vi "DP-Show Noise Floor Data.vi"(1 "Listbox Refnum":refnum<vi>, 9 "Names":string[](array[string]), 11 "error in":errorcluster, 13 "Noise floor data":dbl[][](array[numeric])) -> (15 "error out":errorcluster)   [LabVIEW 2020]
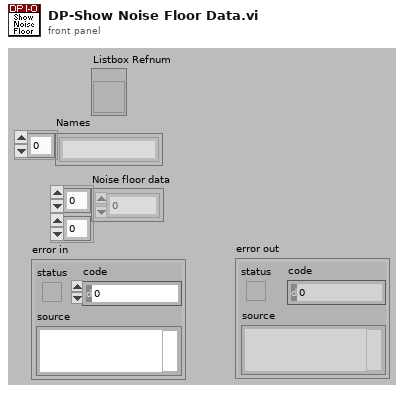
[diagram p1: front panel]
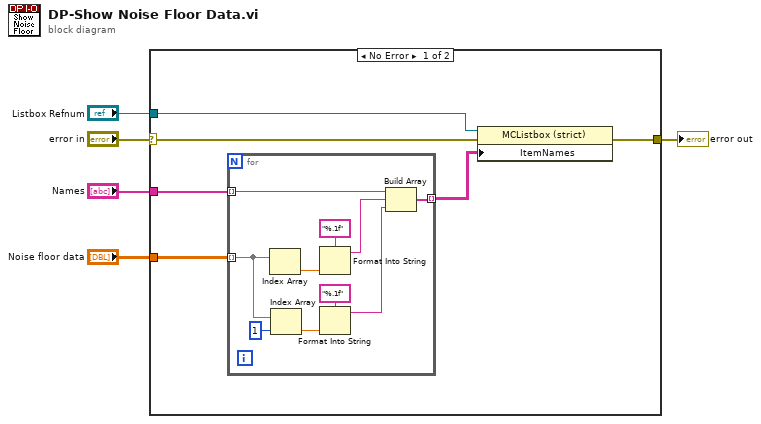
[diagram p0: block diagram]
diagram:
  n1 = case shown="No Error" "error in" {
    selector: "error in" -> [w7 w22]
    tunnel: "Listbox Refnum" -> [w11 _]
    tunnel: "Noise floor data" -> [w10 _]
    tunnel: [w8 w22] -> w3
    tunnel: "Names" -> [w6 _]
    frame No Error {
      n2 = for {
        tunnel: w10 -> [w21] mode=indexing
        tunnel: [w14] -> w9 mode=indexing
        tunnel: w6 -> [w12] mode=indexing
        n3 = Index Array(array=w21) -> (element=w18:dbl)  [unwired: 1 in]
        n4 = Index Array(array=w21, index=1) -> (element=w17:dbl)
        n5 = Format Into String(format string="%.1f", w18) -> (resulting string=w16:string)  [unwired: 2 in, 1 out]
        n6 = Format Into String(format string="%.1f", w17) -> (resulting string=w15:string)  [unwired: 2 in, 1 out]
        n7 = Build Array(w12, w16, w15) -> (w14:string[])
      }
      n8 = property class="MCListbox (strict)"(reference=w11, error in=w7, "ItemNames"=w9) -> (error out=w8:errorcluster)  [unwired: 1 out]
    }
    frame Error {
    }
  }
  "error out" <- w3
